vi "Server Single Connection.vi"() -> ()   [LabVIEW 2013]
doc: "This VI acts as a server for an incoming websockets connection. Receives/sends string data to the connected client."
uses:
  WebSockets/WebSockets.lvlib
panel:
  out "Request URI":string
  out "HTTP Headers":variant
  in  "Stop":bool
  out "Received Data":string
  in  "Send":bool
  in  "Data":string
  # "WebSockets Example"
  # "This VI is a simple example of sending/receiving data using WebSockets.\nIt waits for a single incoming WebSockets connection on Port 6123 and\nthen displays incoming string data. Strings can also be sent back to the client.\n\nInstructions for use:\n1) Run this VI\n2) Open the index.html file located in the examples folder\n3) The index.html will display the status of the connection and once established, data can be sent/received from either this VI or the index.html file."
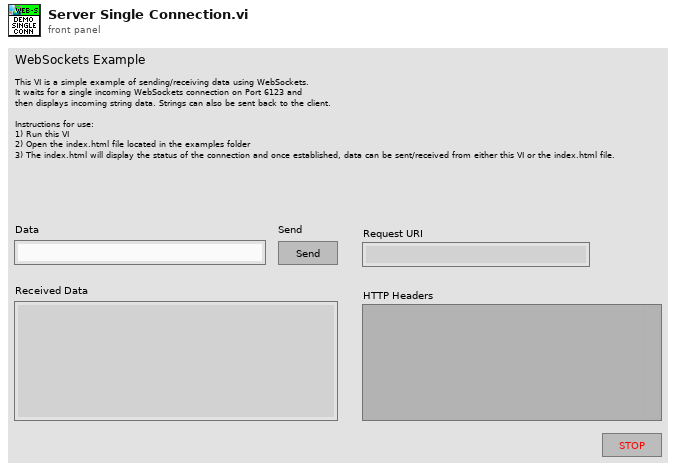
[diagram p1: front panel]
types:
  T1 = typedef "WebSockets.lvlib/Opcodes.ctl" = u8
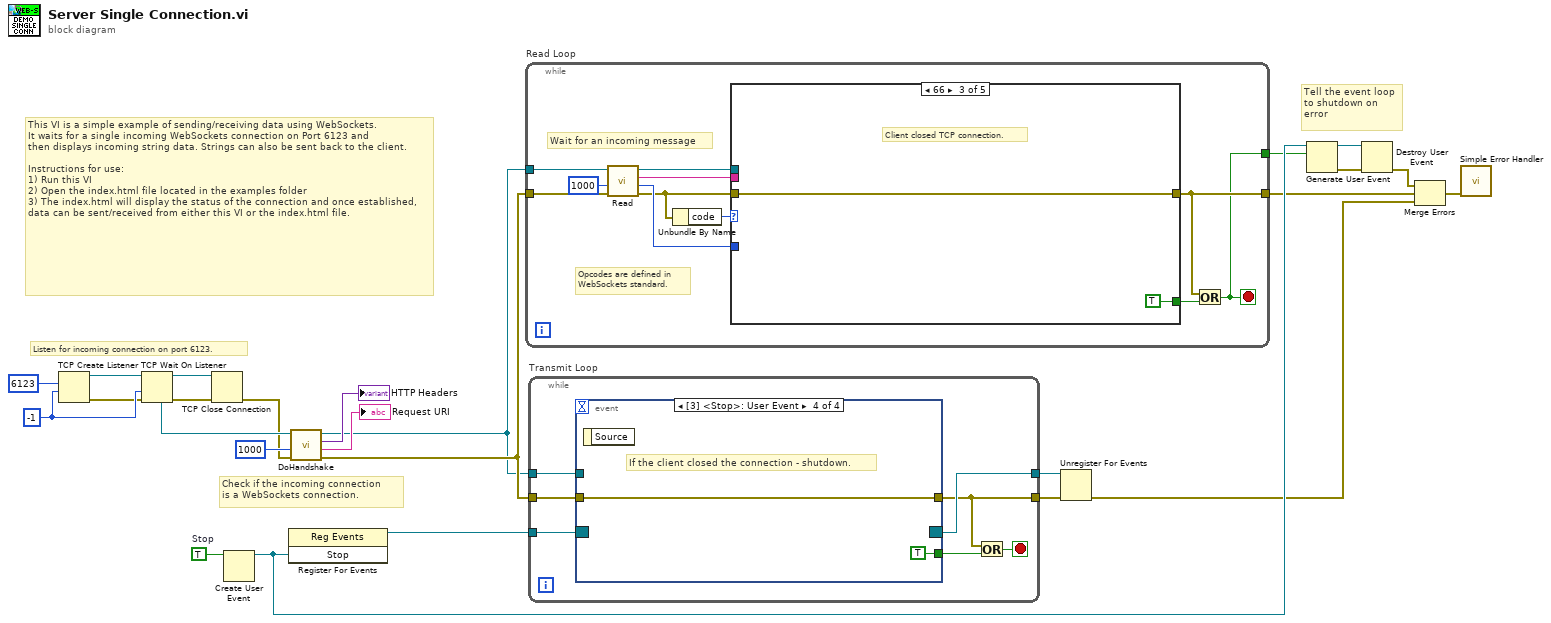
[diagram p0: block diagram]
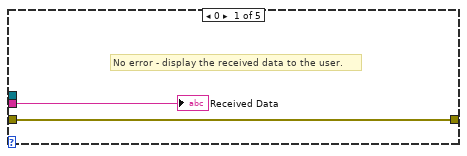
[diagram p2: hidden frame]
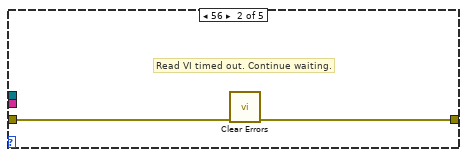
[diagram p3: hidden frame]
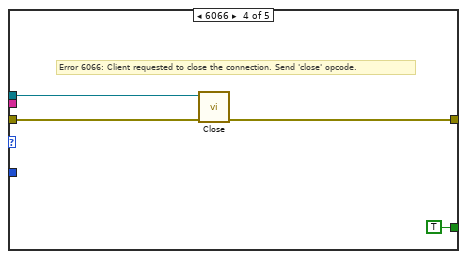
[diagram p4: hidden frame]
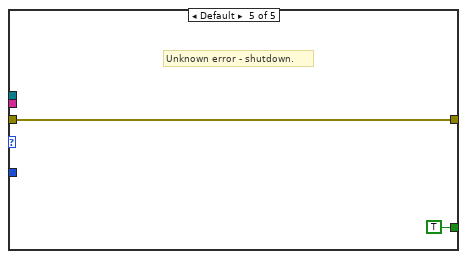
[diagram p5: hidden frame]
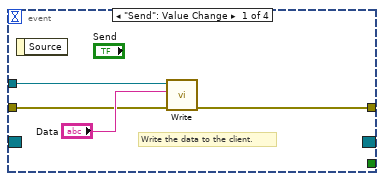
[diagram p6: hidden frame]
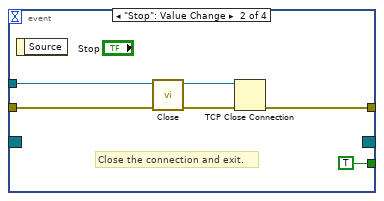
[diagram p7: hidden frame]
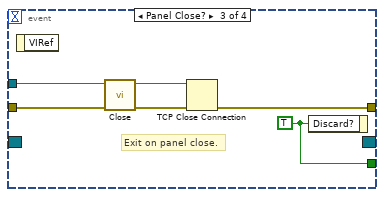
[diagram p8: hidden frame]
diagram:
  w17 = TRUE  # Stop
  w24 = -1 ("timeout ms (25000)")
  # "Tell the event loop to shutdown on error"
  # "This VI is a simple example of sending/receiving data using WebSockets.\nIt waits for a single incoming WebSockets connection on Port 6123 and\nthen displays incoming string data. Strings can also be sent back to the client.\n\nInstructions for use:\n1) Run this VI\n2) Open the index.html file located in the examples folder\n3) The index.html will display the status of the connection and once established, data can be sent/received from either this VI or the index.html file."
  # "Check if the incoming connection\nis a WebSockets connection."
  # "Listen for incoming connection on port 6123."
  n1 = TCP Create Listener(9:w24, 10:u16 6123 ("port")) -> (0:w22:errorcluster, 3:w23:refnum<k5>)  [unwired: 3 in, 1 out]
  n2 = TCP Wait On Listener(8:w22, 9:w24, 11:w23) -> (0:w19:errorcluster, 3:w20:refnum<k5>, 4:w21:refnum<k5>)  [unwired: 1 in, 2 out]
  n3 = TCP Close Connection(connection ID=w20, error in (no error)=w19) -> (error out=w5:errorcluster)  [unwired: 1 in, 1 out]
  n4 = Create User Event(user event datatype=w17) -> (user event=w15:refnum<user-event>)  [unwired: 1 in, 1 out]
  n5 = register-events(w15) -> (reference out=w18:refnum<event-registration>)  [unwired: 2 in, 1 out]
  n6 = call "DoHandshake.vi"("error in (no error)"=w5, "timeout ms (5000)"=1000 ("timeout ms (25000)"), "TCP Connection in"=w21) -> ("error out"=w4:errorcluster, "Request URI"=→"Request URI":string, "Client Headers"=→"HTTP Headers":variant, "WebSocket Server out"=w2:refnum<class "WebSocket Server.lvclass">)  [unwired: 5 in]
  n7 = while "Read Loop" {
    tunnel: w2 -> [w36]
    tunnel: [w26] -> w14
    tunnel: [w28] -> w3
    tunnel: w4 -> [w29]
    stop <- w26 stop-if-true
    # "Wait for an incoming message"
    # "Opcodes are defined in\nWebSockets standard."
    n8 = call "Read.vi"("error in (no error)"=w29, "timeout ms (5000)"=1000 ("timeout ms (25000)"), "WebSocket in"=w36) -> ("error out"=w30:errorcluster, "Opcode"=w31:T1, "Data"=w33:string, "WebSocket out"=w32:refnum<class "WebSocket Server.lvclass">)  [unwired: 4 in, 1 out]
    n9 = Unbundle By Name(w30) -> ("code"=w34:i32)
    n10 = case shown="66" w34 {
      tunnel: w33 -> [w38 _ _ _ _]
      tunnel: [_ _ TRUE TRUE TRUE] -> w27
      tunnel: w32 -> [_ _ _ w46 _]
      tunnel: w31 -> [_ _ _ _ _]
      tunnel: w30 -> [w37 w40 w41 w44 w47]
      tunnel: [w37 w39 w41 w43 w47] -> w28
      frame 0 {
        # "No error - display the received data to the user."
        "Received Data" <- w38
      }
      frame 56 {
        # "Read VI timed out. Continue waiting."
        n11 = call <vilib>:"Clear Errors.vi"("error in (no error)"=w40) -> ("error out"=w39:errorcluster)  [unwired: 6 in]
      }
      frame 66 {
        # "Client closed TCP connection."
      }
      frame 6066 {
        # "Error 6066: Client requested to close the connection. Send 'close' opcode."
        n12 = call "Close.vi"("error in (no error)"=w44, "WebSocket in"=w46) -> ("error out"=w43:errorcluster)  [unwired: 8 in, 1 out]
      }
      frame Default {
        # "Unknown error - shutdown."
      }
    }
    n13 = Or(x=w28, y=w27) -> (x .or. y?=w26:bool)
  }
  n14 = while "Transmit Loop" {
    tunnel: w2 -> [w55]
    tunnel: w18 -> [w54]
    tunnel: [w53] -> w16
    tunnel: [w49] -> w6
    tunnel: w4 -> [w52]
    stop <- w50 stop-if-true
    n15 = event shown="[3] <Stop>: User Event" {
      selector: w54 -> [_ _ _ _]
      dyn-events: [_ _ _ _] -> w53
      timeout: _ -> [_ _ _ _]
      tunnel: w55 -> [w59 w64 w71 _]
      tunnel: [_ TRUE w69 TRUE] -> w51
      tunnel: [w56 w60 w67 w72] -> w49
      tunnel: w52 -> [w57 w61 w66 w72]
      event "Send": Value Change {
        # "Write the data to the client."
        n16 = event-data() -> ()  [unwired: 1 in, 1 out]
        n17 = call "Write.vi"("error in (no error)"=w57, "Data"="Data", "WebSocket in"=w59) -> ("error out"=w56:errorcluster)  [unwired: 7 in, 1 out]
      }
      event "Stop": Value Change {
        # "Close the connection and exit."
        n18 = event-data() -> ()  [unwired: 1 in, 1 out]
        n19 = call "Close.vi"("error in (no error)"=w61, "WebSocket in"=w64) -> ("error out"=w62:errorcluster, "TCP Connection out"=w63:refnum<k5>)  [unwired: 8 in]
        n20 = TCP Close Connection(connection ID=w63, error in (no error)=w62) -> (error out=w60:errorcluster)  [unwired: 1 in, 1 out]
      }
      event Panel Close? {
        w69 = TRUE ("Discard?")
        # "Exit on panel close."
        n21 = event-data() -> ()  [unwired: 1 in, 1 out]
        n22 = call "Close.vi"("error in (no error)"=w66, "WebSocket in"=w71) -> ("error out"=w68:errorcluster, "TCP Connection out"=w70:refnum<k5>)  [unwired: 8 in]
        n23 = TCP Close Connection(connection ID=w70, error in (no error)=w68) -> (error out=w67:errorcluster)  [unwired: 1 in, 1 out]
        n24 = event-data("Discard?"=w69) -> ()  [unwired: 1 in, 1 out]
      }
      event User Event {
        # "If the client closed the connection - shutdown."
        n25 = event-data() -> ()  [unwired: 1 in, 1 out]
      }
    }
    n26 = Or(x=w49, y=w51) -> (x .or. y?=w50:bool)
  }
  n27 = Unregister For Events(event registration refnum=w16, error in=w6) -> (error out=w1:errorcluster)
  n28 = Generate User Event(user event=w15, event data cluster=w14) -> (user event out=w13:refnum<user-event>, error out=w12:errorcluster)  [unwired: 2 in]
  n29 = Destroy User Event(user event=w13, error in=w12) -> (error out=w11:errorcluster)
  n30 = Merge Errors(w11, w3, w1) -> (w7:errorcluster)
  n31 = call <vilib>:"Simple Error Handler.vi"("error in (no error)"=w7) -> ()  [unwired: 4 in, 5 out]
